vi "簇排序.vi"() -> ()   [LabVIEW 2018]
panel:
  in  "簇":T1
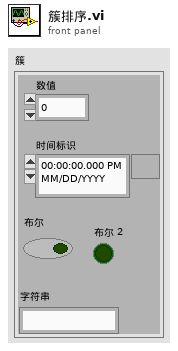
[diagram p1: front panel]
types:
  T1 = cluster{"数值":dbl, "字符串":string, "布尔 2":bool, "布尔":bool, "时间标识":timestamp}
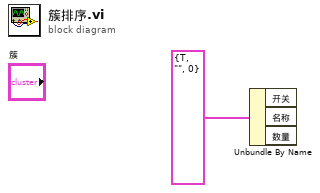
[diagram p0: block diagram]
diagram:
  n1 = Unbundle By Name(cluster{"开关":bool, "名称":string, "数量":i32} {"开关"=TRUE, "名称"="", "数量"=0}) -> ()  [unwired: 3 out]
